vi "data_output_continuous.vi"() -> ()   [LabVIEW 2016]
uses:
  <vilib>/Utility/error.llb/DialogType.ctl
  <vilib>/DAQmx/write.llb/DAQmx Write (Analog 1D Wfm NChan NSamp).vi
  <vilib>/DAQmx/configure/timing.llb/DAQmx Timing (Sample Clock).vi
  <vilib>/DAQmx/create/channels.llb/DAQmx Create Channel (AO-Voltage-Basic).vi
  <vilib>/Analysis/NI_AALPro.lvlib
  <vilib>/Analysis/_algsub.llb/Real Matrix Norm.vi
  <vilib>/DAQmx/create/channels.llb/DAQmx Create Channel (DI-Digital Input).vi
  <resource>/objmgr/daqmx.rc
  <vilib>/DAQmx/read.llb/DAQmx Read (Digital Wfm 1Chan NSamp).vi
  <vilib>/Utility/file.llb/Read Delimited Spreadsheet (DBL).vi
panel:
  out "Digital Waveform Graph":digitalwaveform(graph)
  in  "Stop 2":bool
  in  "Samples per Loop":i32=1000
  in  "Sample Rate 2":dbl=1000.0
  in  "Sample Clock Source 2":tag="PFI0"
  out "Actual Sample Rate":dbl=1000.0 format="%0.2f"
  in  "Line(s)":tag="Dev1/port0/line0:7"
  out "Vector Norm":dbl
  out "Waveform Graph 2":dynamicdata(graph)
  out "Matrix Cols 2":dbl
  out "Matrix Rows 2":dbl
  in  "OK Button":bool
  out "Amplitude":dbl
  in  "Reduce Amplitude":bool
  in  "Sample Rate":dbl=1000.0
  in  "Sample Clock Source":tag="OnboardClock"
  in  "Max Voltage":dbl=5.0
  in  "Min Voltage":dbl=-5.0
  in  "Physical Channel(s)":tag="Dev1/ao0"
  in  "Stop":bool
  out "Number of Samples Written per Channel":dbl
  out "Waveform Graph":dynamicdata(graph)
  out "Matrix Cols":dbl
  out "Matrix Rows":dbl
  in  "csv Path":path
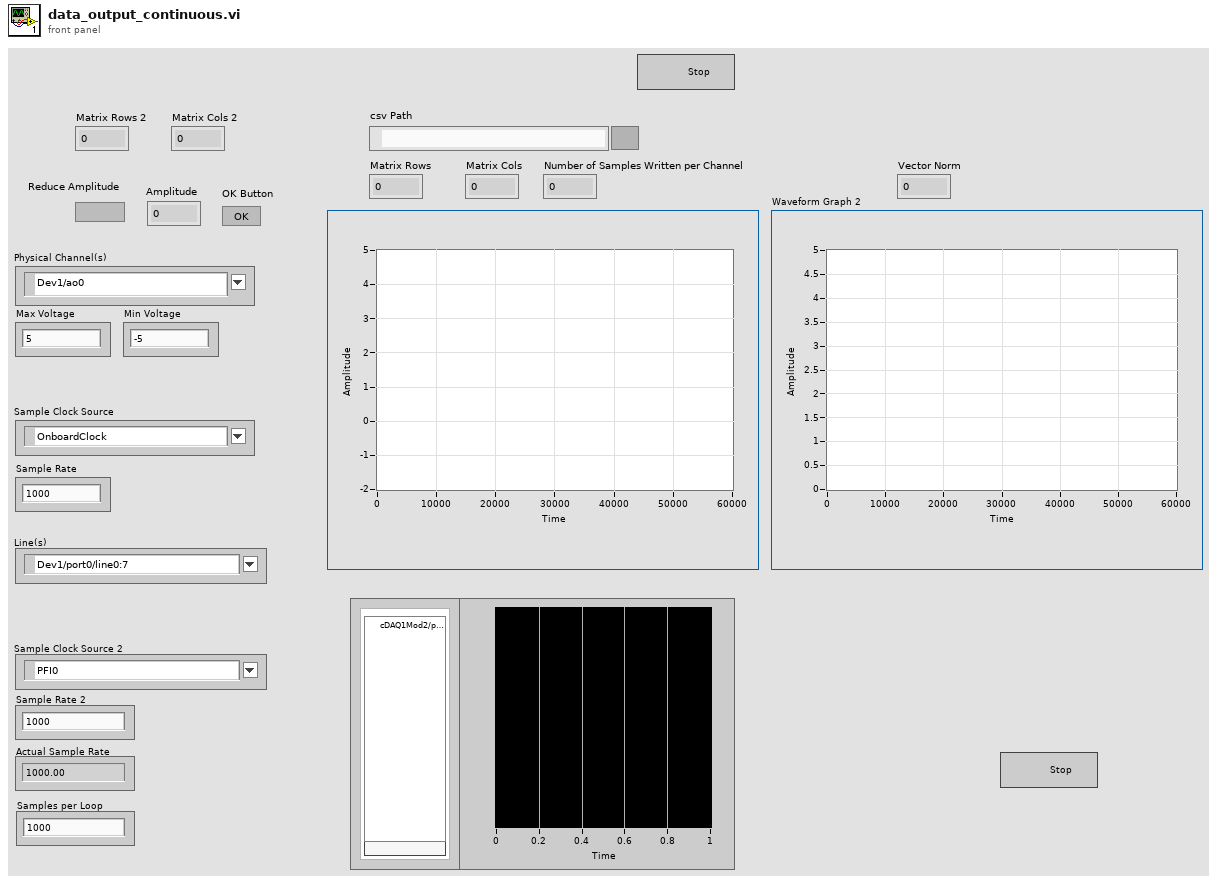
[diagram p1: front panel]
types:
  T1 = typedef "DialogType.ctl" = u16
  T2 = typedef "NI_Matrix.lvlib/RealMatrix.ctl" = dbl[][]
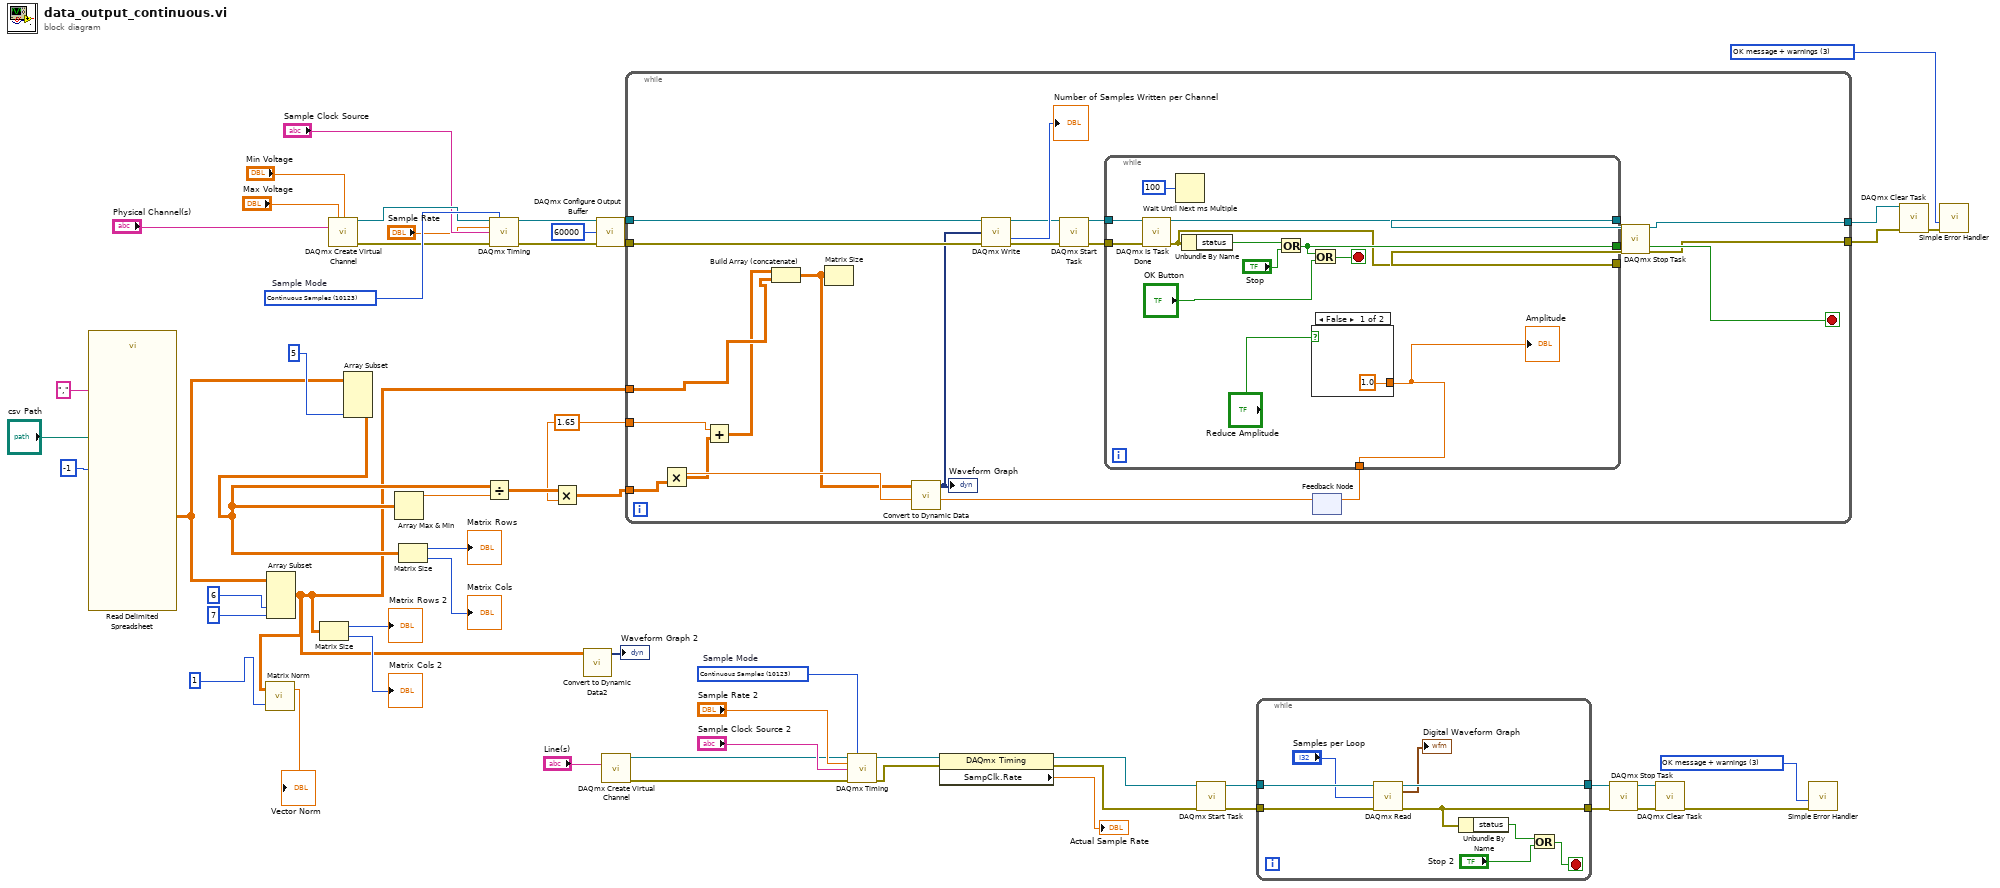
[diagram p0: block diagram]
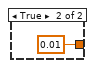
[diagram p2: hidden frame]
diagram:
  w3 = T1 3 items=["no dialog", "OK message", "continue or stop message", "OK message + warnings", "continue/stop + warnings"] ("type of dialog (OK msg:1)")
  w18 = 10123 items=["Finite Samples"=10178, "Continuous Samples"=10123, "Hardware Timed Single Point"=12522]  # Sample Mode
  w47 = 10123 items=["Finite Samples"=10178, "Continuous Samples"=10123, "Hardware Timed Single Point"=12522]  # Sample Mode
  w48 = T1 3 items=["no dialog", "OK message", "continue or stop message", "OK message + warnings", "continue/stop + warnings"] ("type of dialog (OK msg:1)")
  w20 = 1.65
  n1 = call-poly <vilib>:"Read Delimited Spreadsheet.vi"("file path (dialog if empty)"="csv Path", "number of rows (all:-1)"=-1, "delimiter (\\t)"=",") -> ("all rows"=w30:dbl[][])  [unwired: 7 in, 5 out]
  n2 = Array Subset(array=w30, index (col)=6, length (col)=7) -> (w24:dbl[][])  [unwired: 2 in]
  n3 = call-poly <vilib>:"Matrix Norm.vi"("norm type"=1, "Input Matrix"=w24) -> ("norm"=→"Vector Norm":dbl)  [unwired: 1 out]
  n4 = Matrix Size(0:w24) -> (1:→"Matrix Rows 2":i32, 2:→"Matrix Cols 2":i32)
  n5 = call-poly <vilib>:"DAQmx Create Virtual Channel.vi"("maximum value"="Max Voltage", "minimum value"="Min Voltage", "physical channels"="Physical Channel(s)") -> ("task out"=w45:refnum<k21>, "error out"=w46:errorcluster)  [unwired: 11 in]
  n6 = Array Subset(array=w30, length (col)=5) -> (w32:dbl[][])  [unwired: 3 in]
  n7 = Array Max & Min(array=w32) -> (max value=w53:dbl)  [unwired: 3 out]
  n8 = Matrix Size(0:w32) -> (1:→"Matrix Rows":i32, 2:→"Matrix Cols":i32)
  n9 = Divide(x=w32, y=w53) -> (x/y=w52:dbl[][])
  n10 = call-poly <vilib>:"DAQmx Timing.vi"("task/channels in"=w45, "sample mode"=w47, "rate"="Sample Rate", "source"="Sample Clock Source", "error in"=w46) -> ("task out"=w39:refnum<k21>, "error out"=w37:errorcluster)  [unwired: 9 in]
  n11 = Multiply(x=w52, y=w20) -> (x*y=w21:dbl[][])
  n12 = call "Convert to Dynamic Data2"("2D Array"=w24) -> ("Dynamic Data Type"=→"Waveform Graph 2":dynamicdata)  [unwired: 3 in]
  n13 = call <vilib>:"DAQmx Configure Output Buffer.vi"("task/channels in"=w39, "buffer size (in samples per channel)"=60000, "error in"=w37) -> ("task out"=w36:refnum<k21>, "error out"=w35:errorcluster)  [unwired: 11 in]
  n14 = call-poly <vilib>:"DAQmx Create Virtual Channel.vi"("lines"="Line(s)") -> ("task out"=w15:refnum<k21>, "error out"=w14:errorcluster)  [unwired: 13 in]
  n15 = while {
    tunnel: w36 -> [w72]
    tunnel: w35 -> [w71]
    tunnel: w21 -> [w68]
    tunnel: [w64] -> w34
    tunnel: [w63] -> w33
    tunnel: w24 -> [w61]
    tunnel: w20 -> [w59]
    stop <- w69 stop-if-true
    n16 = feedback #1() -> (w67:dbl)  [unwired: 1 in]
    n17 = Multiply(x=w67, y=w68) -> (x*y=w57:dbl[][])
    n18 = Add(x=w59, y=w57) -> (x+y=w58:dbl[][])
    n19 = Build Array (concatenate)(w58, w61) -> (w60:T2)
    n20 = Matrix Size(0:w60) -> ()  [unwired: 2 out]
    n21 = call "Convert to Dynamic Data"("2D Array"=w60) -> ("Dynamic Data Type"=w70:dynamicdata)  [unwired: 3 in]
    "Waveform Graph" <- w70
    n22 = call-poly <vilib>:"DAQmx Write.vi"("task/channels in"=w72, "data"=w70, "error in"=w71) -> ("task out"=w76:refnum<k21>, "number of samples written per channel"=→"Number of Samples Written per Channel":u32, "error out"=w75:errorcluster)  [unwired: 10 in]
    n23 = call <vilib>:"DAQmx Start Task.vi"("task/channels in"=w76, "error in"=w75) -> ("task out"=w73:refnum<k21>, "error out"=w74:errorcluster)  [unwired: 12 in]
    n24 = while {
      tunnel: w73 -> [w86]
      tunnel: w74 -> [w85]
      tunnel: [w83] -> w69
      tunnel: [w82] -> w66
      tunnel: [w81] -> w65
      tunnel: [w78] -> w62
      stop <- w84 stop-if-true
      n25 = call <vilib>:"DAQmx Is Task Done.vi"("task/channels in"=w86, "error in"=w85) -> ("task out"=w82:refnum<k21>, "error out"=w81:errorcluster)  [unwired: 11 in, 1 out]
      n26 = Wait Until Next ms Multiple(millisecond multiple=u32 100) -> ()  [unwired: 1 out]
      n27 = Unbundle By Name(w81) -> ("status"=w89:bool)
      n28 = Or(x=w89, y="Stop") -> (x .or. y?=w83:bool)
      n29 = Or(x=w83, y="OK Button") -> (x .or. y?=w84:bool)
      n30 = case shown="False" "Reduce Amplitude" {
        tunnel: [1.0 0.01] -> w78
        frame False {
        }
        frame True {
        }
      }
      "Amplitude" <- w78
    }
    n31 = feedback-in #1(w62) -> ()
    n32 = call <vilib>:"DAQmx Stop Task.vi"("task/channels in"=w66, "error in"=w65) -> ("task out"=w64:refnum<k21>, "error out"=w63:errorcluster)  [unwired: 12 in]
  }
  n33 = call-poly <vilib>:"DAQmx Timing.vi"("task/channels in"=w15, "sample mode"=w18, "rate"="Sample Rate 2", "source"="Sample Clock Source 2", "error in"=w14) -> ("task out"=w13:refnum<k21>, "error out"=w12:errorcluster)  [unwired: 9 in]
  n34 = property class="DAQmx Timing"(reference=w13, error in=w12) -> (reference out=w2:refnum<k21>, error out=w1:errorcluster, "SampClk.Rate"=→"Actual Sample Rate":dbl)
  n35 = call <vilib>:"DAQmx Start Task.vi"("task/channels in"=w2, "error in"=w1) -> ("task out"=w8:refnum<k21>, "error out"=w9:errorcluster)  [unwired: 12 in]
  n36 = while {
    tunnel: [w100] -> w5
    tunnel: [w96] -> w4
    tunnel: w9 -> [w99]
    tunnel: w8 -> [w98]
    stop <- w93 stop-if-true
    n37 = call-poly <vilib>:"DAQmx Read.vi"("task/channels in"=w98, "number of samples per channel"="Samples per Loop", "error in"=w99) -> ("task out"=w100:refnum<k21>, "data"=→"Digital Waveform Graph":digitalwaveform, "error out"=w96:errorcluster)  [unwired: 10 in]
    n38 = Unbundle By Name(w96) -> ("status"=w95:bool)
    n39 = Or(x=w95, y="Stop 2") -> (x .or. y?=w93:bool)
  }
  n40 = call <vilib>:"DAQmx Stop Task.vi"("task/channels in"=w5, "error in"=w4) -> ("task out"=w7:refnum<k21>, "error out"=w6:errorcluster)  [unwired: 12 in]
  n41 = call <vilib>:"DAQmx Clear Task.vi"("task in"=w7, "error in"=w6) -> ("error out"=w10:errorcluster)  [unwired: 13 in]
  n42 = call <vilib>:"Simple Error Handler.vi"("type of dialog (OK msg:1)"=w3, "error in (no error)"=w10) -> ()  [unwired: 3 in, 5 out]
  n43 = call <vilib>:"DAQmx Clear Task.vi"("task in"=w34, "error in"=w33) -> ("error out"=w49:errorcluster)  [unwired: 13 in]
  n44 = call <vilib>:"Simple Error Handler.vi"("type of dialog (OK msg:1)"=w48, "error in (no error)"=w49) -> ()  [unwired: 3 in, 5 out]
